vi "snake.vi"() -> ()   [LabVIEW 2021]
uses:
  <vilib>/Utility/inputDevices.llb/keyboardAcquire.vi
  <vilib>/Utility/inputDevices.llb/closeKeyboard.vi
panel:
  out "Array":bool[][](array[boolean])
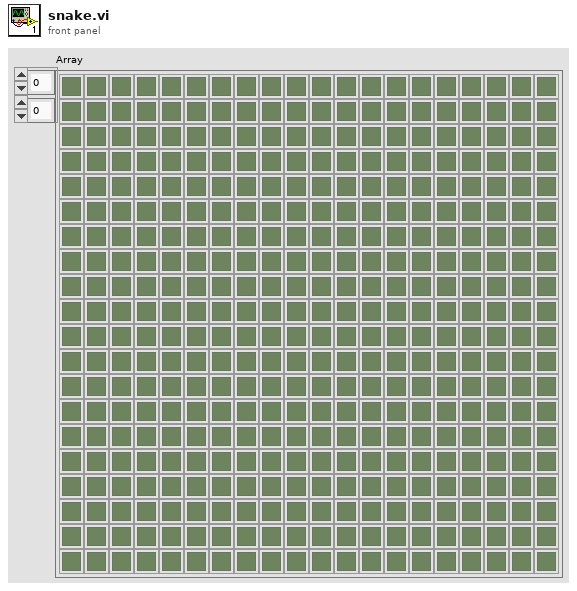
[diagram p1: front panel]
types:
  T1 = enum16{"0", "1", "2", "3", "4", "5", "6", "7", "8", "9", "A", "B", "C", "D", "E", "F", "G", "H", "I", "J", "K", "L", "M", "N", "O", "P", "Q", "R", "S", "T", "U", "V", "W", "X", "Y", "Z", "F1", "F2", "F3", "F4", "F5", "F6", "F7", "F8", "F9", "F10", "F11", "F12", "F13", "F14", "F15", "ADD", "BACK", "BACKSLASH", "CAPITAL", "COMMA", "DECIMAL", "DELETE", "DIVIDE", "DOWN", "END", "EQUALS", "ESCAPE", "GRAVE (`)", "HOME", "INSERT", "LBRACKET", "LCONTROL", "LEFT", "L ALT", "LSHIFT", "LWIN", "MINUS", "MULTIPLY", "NEXT", "NUMLOCK", "NUMPAD_0", "NUMPAD_1", "NUMPAD_2", "NUMPAD_3", "NUMPAD_4", "NUMPAD_5", "NUMPAD_6", "NUMPAD_7", "NUMPAD_8", "NUMPAD_9", "PAUSE", "PERIOD", "PRIOR (PG UP)", "RBRACKET", "RCONTROL", "RETURN", "RIGHT", "R ALT", "RSHIFT", "RWIN", "SCROLL", "SEMICOLON", "SLASH", "SPACE", "SUBTRACT", "TAB", "UP", "ENTER (num pad)", "' (quote)"}[]
  T2 = enum16{"0", "1", "2", "3", "4", "5", "6", "7", "8", "9", "A", "B", "C", "D", "E", "F", "G", "H", "I", "J", "K", "L", "M", "N", "O", "P", "Q", "R", "S", "T", "U", "V", "W", "X", "Y", "Z", "F1", "F2", "F3", "F4", "F5", "F6", "F7", "F8", "F9", "F10", "F11", "F12", "F13", "F14", "F15", "ADD", "BACK", "BACKSLASH", "CAPITAL", "COMMA", "DECIMAL", "DELETE", "DIVIDE", "DOWN", "END", "EQUALS", "ESCAPE", "GRAVE (`)", "HOME", "INSERT", "LBRACKET", "LCONTROL", "LEFT", "L ALT", "LSHIFT", "LWIN", "MINUS", "MULTIPLY", "NEXT", "NUMLOCK", "NUMPAD_0", "NUMPAD_1", "NUMPAD_2", "NUMPAD_3", "NUMPAD_4", "NUMPAD_5", "NUMPAD_6", "NUMPAD_7", "NUMPAD_8", "NUMPAD_9", "PAUSE", "PERIOD", "PRIOR (PG UP)", "RBRACKET", "RCONTROL", "RETURN", "RIGHT", "R ALT", "RSHIFT", "RWIN", "SCROLL", "SEMICOLON", "SLASH", "SPACE", "SUBTRACT", "TAB", "UP", "ENTER (num pad)", "' (quote)"}
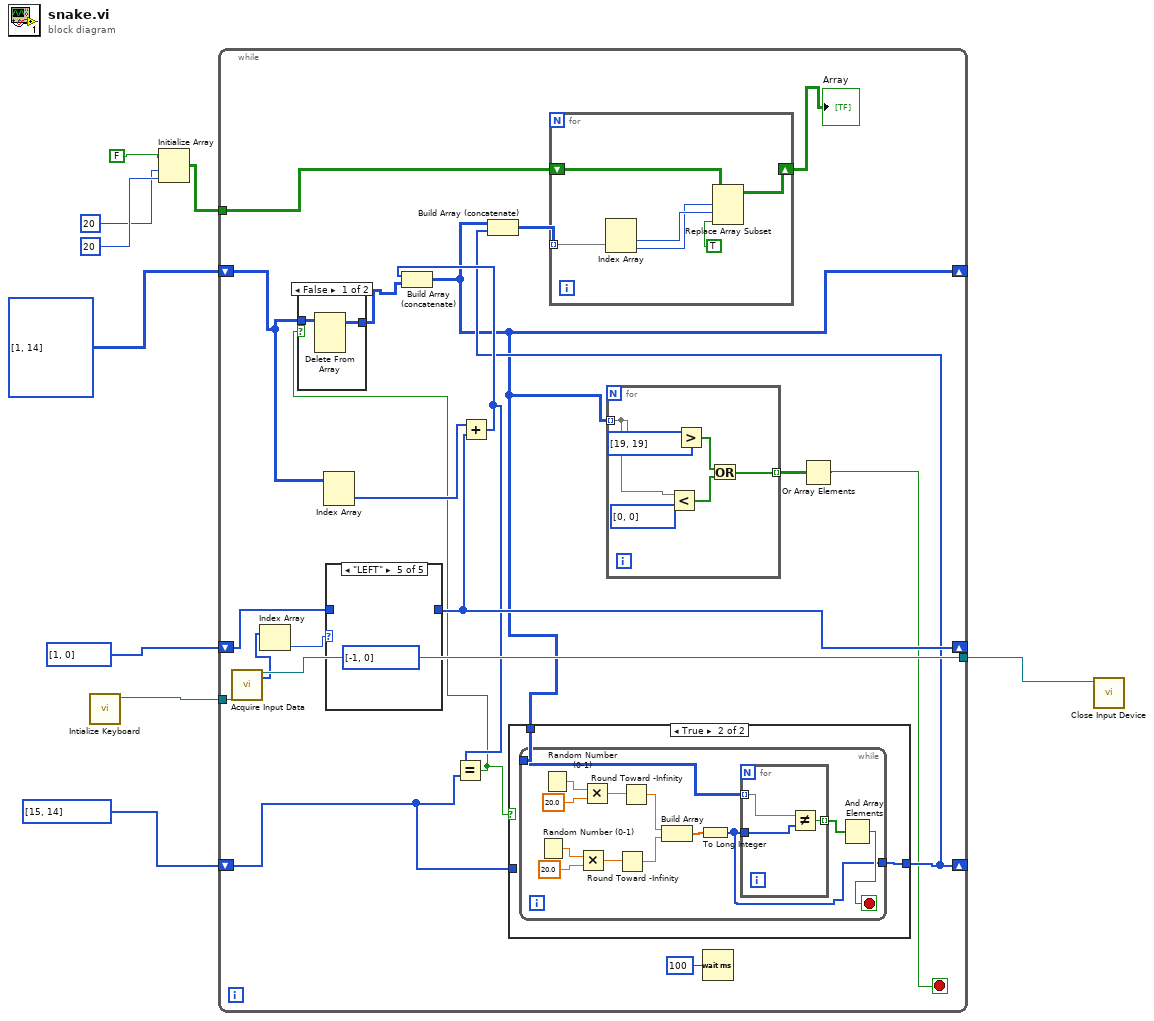
[diagram p0: block diagram]
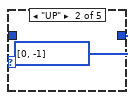
[diagram p5: hidden frame]
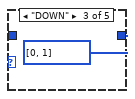
[diagram p6: hidden frame]
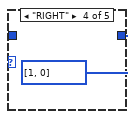
[diagram p7: hidden frame]
diagram:
  n1 = call <vilib>:"Intialize Keyboard.vi"() -> ("device ID"=w4:refnum<k1>)  [unwired: 10 in, 1 out]
  n2 = Initialize Array(FALSE, 20, 20) -> (w7:bool[][])
  n3 = while {
    tunnel: w7 -> [w25]
    tunnel: [w28] -> w5
    tunnel: w4 -> [w27]
    shift-right: [w21] -> _
    shift-left: i32[] [1, 0] -> [w23]
    shift-right: [w12] -> _
    shift-left: i32[][] [[1, 14]] -> [w20]
    shift-right: [w13] -> _
    shift-left: i32[] [15, 14] -> [w15]
    stop <- w10 stop-if-true
    n4 = call-poly <vilib>:"Acquire Input Data.vi"("device ID"=w27) -> ("device ID"=w28:refnum<k1>, "keys pressed"=w26:T1)  [unwired: 16 in, 1 out]
    n5 = Index Array(array=w26) -> (element=w18:T2)  [unwired: 1 in]
    n6 = Index Array(array=w20) -> (element=w22:i32[])  [unwired: 2 in]
    n7 = case shown="\"LEFT\"" w18 {
      tunnel: w23 -> [w58 _ _ _ _]
      tunnel: [w58 i32[] [0, -1] i32[] [0, 1] i32[] [1, 0] i32[] [-1, 0]] -> w21
      frame Default {
      }
      frame "UP" {
      }
      frame "DOWN" {
      }
      frame "RIGHT" {
      }
      frame "LEFT" {
      }
    }
    n8 = Add(x=w22, y=w21) -> (x+y=w17:i32[])
    n9 = Equal?(x=w17, y=w15) -> (x = y?=w16:bool)
    n10 = case shown="False" w16 {
      tunnel: w20 -> [w56 w57]
      tunnel: [w55 w57] -> w19
      frame False {
        n11 = Delete From Array(array=w56) -> (array with subset deleted=w55:i32[][])  [unwired: 3 in, 1 out]
      }
      frame True {
      }
    }
    n12 = Build Array (concatenate)(w17, w19) -> (w12:i32[][])
    n13 = case shown="True" w16 {
      tunnel: w12 -> [_ w38]
      tunnel: [w36 w37] -> w13
      tunnel: w15 -> [w36 _]
      frame False {
      }
      frame True {
        n14 = while {
          tunnel: w38 -> [w42]
          tunnel: [w39] -> w37
          stop <- w40 stop-if-true
          n15 = Random Number (0-1)() -> (number: 0 to 1=w48:dbl)
          n16 = Random Number (0-1)() -> (number: 0 to 1=w51:dbl)
          n17 = Multiply(x=w48, y=20.0 ("x")) -> (x*y=w46:dbl)
          n18 = Multiply(x=w51, y=20.0 ("x")) -> (x*y=w49:dbl)
          n19 = Round Toward -Infinity(1:w46) -> (0:w44:dbl)
          n20 = Round Toward -Infinity(1:w49) -> (0:w45:dbl)
          n21 = Build Array(w45, w44) -> (w43:dbl[])
          n22 = To Long Integer(number=w43) -> (32bit integer=w39:i32[])
          n23 = for {
            tunnel: w42 -> [w54] mode=indexing
            tunnel: w39 -> [w53]
            tunnel: [w52] -> w41 mode=indexing
            n24 = Not Equal?(x=w54, y=w53) -> (x != y?=w52:bool)
          }
          n25 = And Array Elements(Boolean array=w41) -> (logical AND=w40:bool)
        }
      }
    }
    n26 = Build Array (concatenate)(w12, w13) -> (w14:i32[][])
    n27 = for {
      shift-right: [w67] -> w24
      shift-left: w25 -> [w68]
      tunnel: w14 -> [w66] mode=indexing
      n28 = Index Array(array=w66) -> (element #1=w65:i32, element #2=w64:i32)  [unwired: 2 in]
      n29 = Replace Array Subset(array=w68, new element=TRUE, index (row)=w64, index (col)=w65) -> (w67:bool[][])
    }
    "Array" <- w24
    n30 = for {
      tunnel: w12 -> [w34] mode=indexing
      tunnel: [w31] -> w11 mode=indexing
      n31 = Less?(x=w34, y=i32[] [0, 0] ("x")) -> (x < y?=w32:bool[])
      n32 = Greater?(x=w34, y=i32[] [19, 19]) -> (0:w33:bool[])
      n33 = Or(x=w33, y=w32) -> (x .or. y?=w31:bool[])
    }
    n34 = Wait (ms)(milliseconds to wait=u32 100) -> ()  [unwired: 1 out]
    n35 = Or Array Elements(Boolean array=w11) -> (logical OR=w10:bool)
  }
  n36 = call-poly <vilib>:"Close Input Device.vi"("device ID"=w5) -> ()  [unwired: 9 in, 1 out]
